vi "Scrub.vi"(8 "error in":errorcluster, 10 "Input String":string, 11 "Date Scrubber in":refnum<class "Date Scrubber.lvclass">) -> (0 "error out":errorcluster, 2 "Scrubbed String":string, 3 "Date Scrubber out":refnum<class "Date Scrubber.lvclass">)   [LabVIEW 2020, in "Approval Tests.lvlib" / "Date Scrubber.lvclass"]
uses:
  Date Scrubber.lvclass
  Date Scrubber.lvclass/Date Scrubber.ctl
  Regex Scrubber Count Unique/Regex Scrubber Count Unique.lvclass
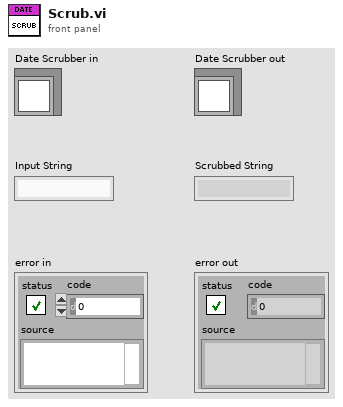
[diagram p1: front panel]
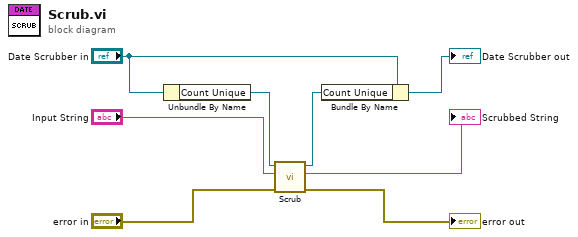
[diagram p0: block diagram]
diagram:
  n1 = Unbundle By Name("Date Scrubber in") -> ("Count Unique"=w4:refnum<class "Regex Scrubber Count Unique.lvclass">)
  n2 = call-dynamic "Scrub.vi"("error in"="error in", "Input String"="Input String", "Regex Scrubber in"=w4) -> ("error out"=→"error out":errorcluster, "Scrubbed String"=→"Scrubbed String":string, "Regex Scrubber out"=w3:refnum<class "Regex Scrubber Count Unique.lvclass">)  [unwired: 6 in]
  n3 = Bundle By Name(cluster="Date Scrubber in", "Count Unique"=w3) -> (→"Date Scrubber out":refnum<class "Date Scrubber.lvclass">)
